vi "FSK_Judgement.vi"(8 "error in (no error)":errorcluster caption="错误输入（无错误）", 10 "RecvDeSync":dbl[](array[numeric]), 11 "PathIn":path) -> (0 "error out":errorcluster caption="错误输出", 2 "judgeSampled_data":dbl[](array[numeric]) format="%#_13g", 3 "PathOut":path)   [LabVIEW 2015]
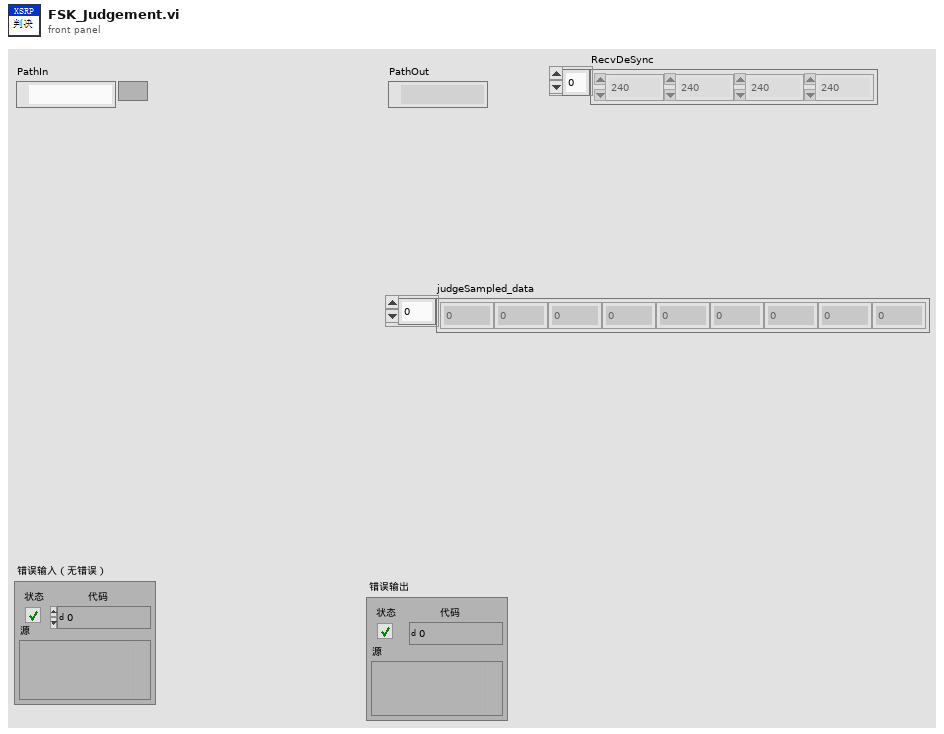
[diagram p1: front panel]
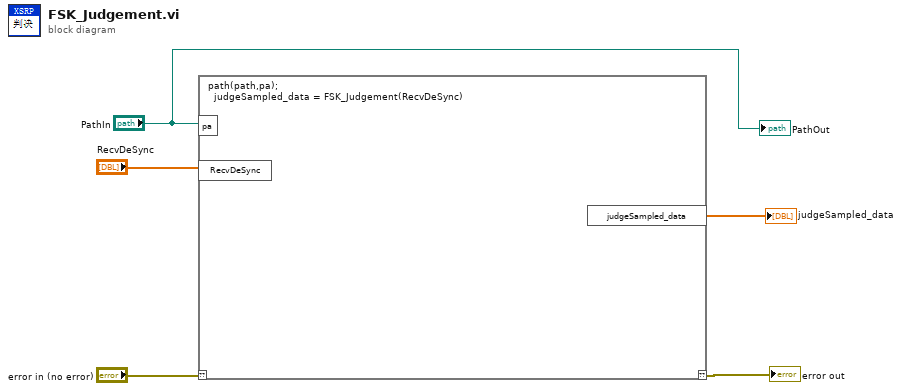
[diagram p0: block diagram]
diagram:
  n1 = script code="path(path,pa);\n  judgeSampled_data = FSK_Judgement(RecvDeSync)"("??"="error in (no error)", "pa"="PathIn", "RecvDeSync"="RecvDeSync") -> ("??"=→"error out":errorcluster, "judgeSampled_data"=→"judgeSampled_data":dbl[])
  "PathOut" <- "PathIn"
